vi "Page - Ports.vi"(8 "error in (no error)":errorcluster, 11 "Node Ptr":T3 format="%.0x") -> (0 "error out":errorcluster)   [LabVIEW 2015, in "SLSC-12201 DIO System Explorer.lvlib"]
uses:
  SLSC-12201 DIO System Explorer.lvlib
  <vilib>/NI Veristand/Custom Device API/Custom Device Item Ref.ctl
  <vilib>/Utility/miscctls.llb/LVRowAndColumnTypeDef.ctl
  Direction Control.ctl
  Shared/Constants.vi
  <vilib>/NI Veristand/Custom Device API/Custom Device API.lvlib
  Shared/SLSC-12201 DIO Shared.lvlib
panel:
  in  "Apply":bool
  in  "Port Type":T1 items=["Input", "Output Source", "Output Sink", "Output Push-Pull"]
  out "Cell Position":T2
  in  "Type":u16(ring) items=["Input", "Output Source", "Output Sink", "Output Pull-up"]
  out "Multicolumn Listbox":i32(listbox)=4
  in  "Disable Port":bool
  in  "Enable Port":bool
  in  "SHDocVw.IWebBrowser2":refnum<k7>(container)
  in  "Header":cluster{"Section Name":string}={"Section Name"="Custom Device Item Settings"}
  in  "Description":string
  out "Name":string
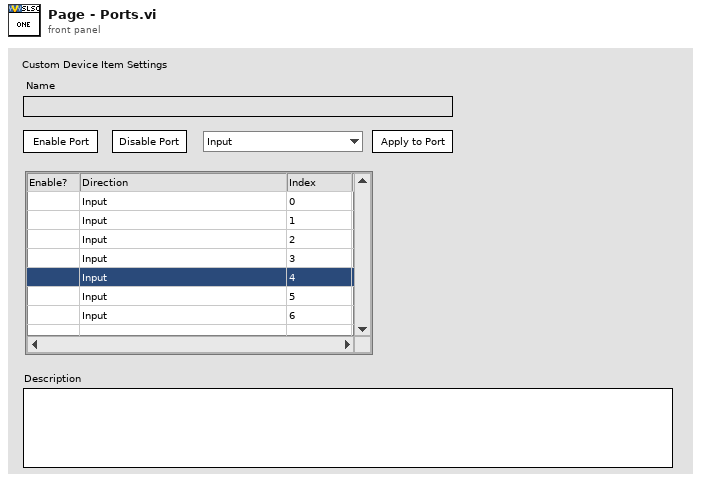
[diagram p1: front panel]
types:
  T1 = typedef "SLSC-12201 DIO System Explorer.lvlib/Direction Control.ctl" = u16
  T2 = typedef "LVRowAndColumnTypeDef.ctl" = cluster{"Row":i32, "Column":i32}
  T3 = typedef "Custom Device API.lvlib/Custom Device Item Ref.ctl" = u64
  T4 = typedef "Custom Device API.lvlib/Custom Device Item Info.ctl" = cluster{"Name":string, "Is Channel":bool, "GUID":string, "Is Waveform":bool}
  T5 = typedef "Custom Device API.lvlib/Custom Device Channel.ctl" = cluster{"Type":T6, "Units":string, "Default Value":dbl, "Faultable":bool, "Scalable":bool}
  T6 = typedef "Custom Device API.lvlib/Custom Device Channel Type.ctl" = enum16{"Input", "Output"}
  T7 = cluster{"Channel Name":string, "SLSC Name":string, "Channel":T5}[]
  T8 = typedef "Custom Device API.lvlib/Custom Device Commands.ctl" = enum16{"Default", "Item renamed", "Shutdown", "Dynamic button pressed"}
  T9 = typedef "LVPoint32TypeDef.ctl" = cluster{"Horizontal":i32, "Vertical":i32}
  T10 = typedef "LVPositionTypeDef.ctl" = cluster{"Left":i32, "Top":i32}
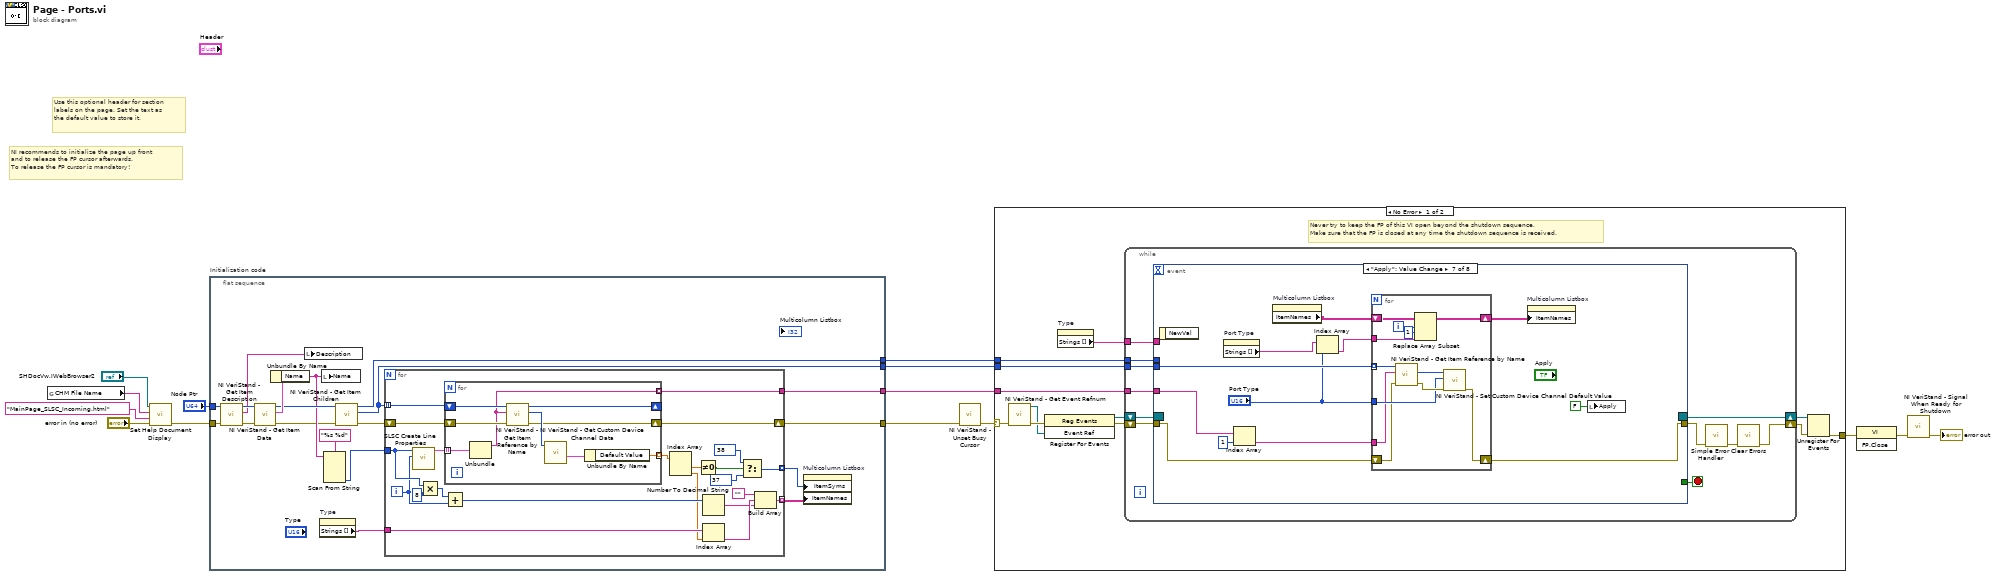
[diagram p0: block diagram]
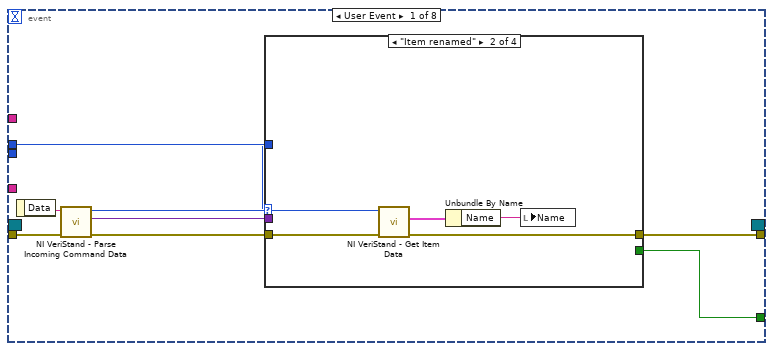
[diagram p2: hidden frame]
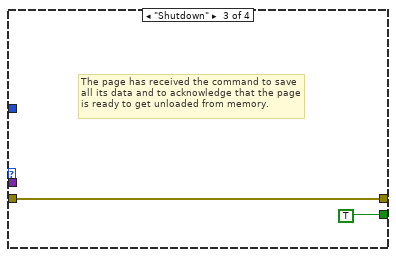
[diagram p4: hidden frame]
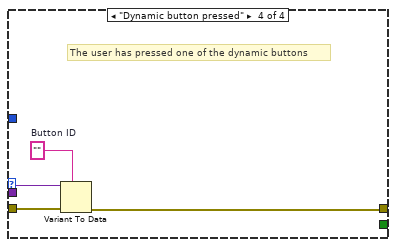
[diagram p5: hidden frame]
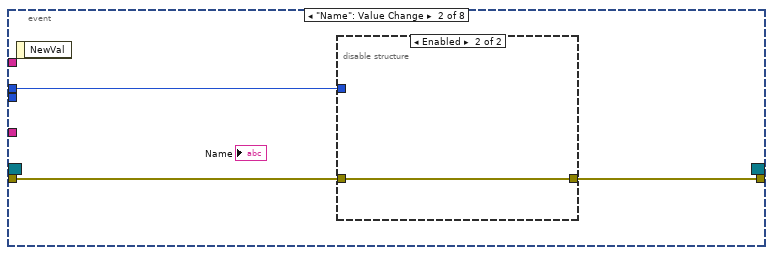
[diagram p6: hidden frame]
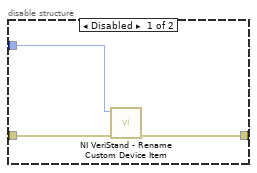
[diagram p7: hidden frame]
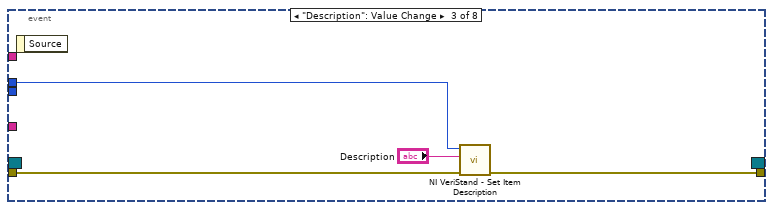
[diagram p8: hidden frame]
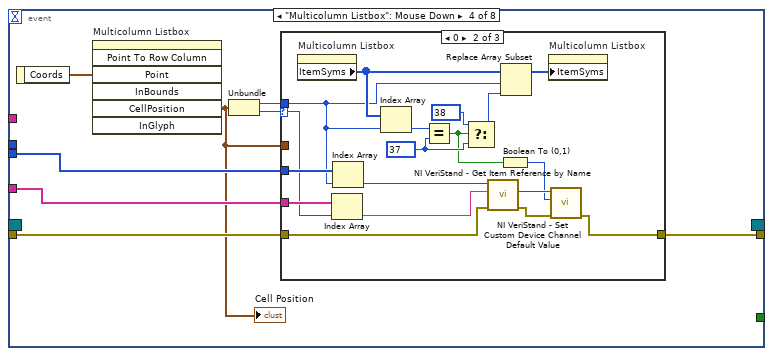
[diagram p9: hidden frame]
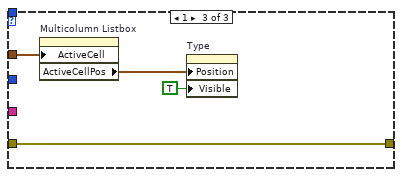
[diagram p11: hidden frame]
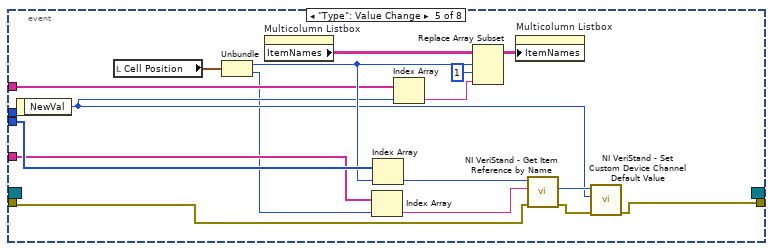
[diagram p12: hidden frame]
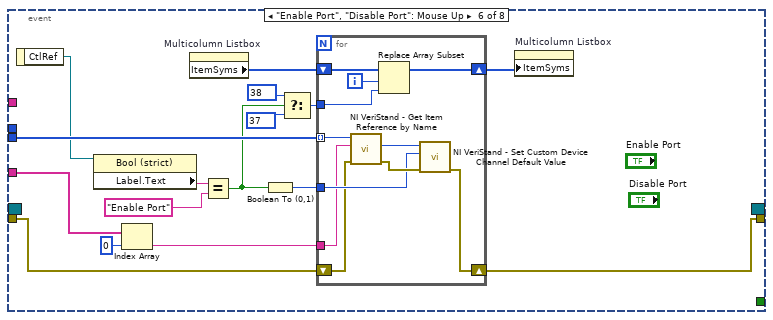
[diagram p13: hidden frame]
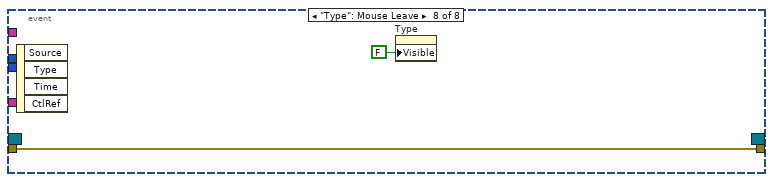
[diagram p14: hidden frame]
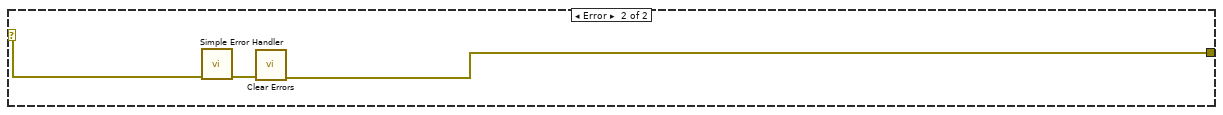
[diagram p15: hidden frame]
diagram:
  # "Use this optional header for section labels on the page. Set the text as the default value to store it."
  # "NI recommends to initialize the page up front\nand to release the FP cursor afterwards.\nTo release the FP cursor is mandatory!"
  n1 = global read "Constants.vi" "CHM File Name"() -> (w3:string)
  n2 = call "Set Help Document Display.vi"("error in (no error)"="error in (no error)", "HTML File"="MainPage_SLSC_Incoming.html", "Main CHM File"=w3, "SHDocVw.IWebBrowser2"="SHDocVw.IWebBrowser2") -> ("error out"=w4:errorcluster)  [unwired: 7 in]
  n3 = flat-sequence "Initialization code" {
    tunnel: w4 -> [w32]
    tunnel: "Node Ptr" -> [w31]
    tunnel: [w27] -> w10
    tunnel: [w25] -> w8
    tunnel: [w21] -> w2
    tunnel: [w20] -> w1
    frame #0 {
      n4 = call <vilib>:"NI VeriStand - Get Item Description.vi"("error in (no error)"=w32, "Item Ref in"=w31) -> ("error out"=w29:errorcluster, "Description"=w30:string, "Item Ref out"=w33:T3)  [unwired: 7 out]
      n5 = call <vilib>:"NI VeriStand - Get Item Data.vi"("error in (no error)"=w29, "Item Ref in"=w33) -> ("error out"=w19:errorcluster, "Item Info"=w28:T4, "Item Ref out"=w26:T3)  [unwired: 7 out]
      n6 = Unbundle By Name(w28) -> ("Name"=w23:string)
      n7 = local write "Description"(w30) -> ()
      n8 = property on="Type" class="Ring (strict)"() -> ("Strings []"=w17:string[])  [unwired: 2 in, 2 out]
      n9 = local write "Name"(w23) -> ()
      n10 = Scan From String(format string="%s %d", input string=w23) -> (output 2=w22:i32)  [unwired: 5 in, 3 out]
      n11 = call <vilib>:"NI VeriStand - Get Item Children.vi"("error in (no error)"=w19, "Item Ref in"=w26) -> ("error out"=w18:errorcluster, "Child Refs"=w21:T3[], "Item Ref out"=w25:T3)  [unwired: 6 in, 1 out]
      n12 = for {
        shift-right: [w54] -> w27
        shift-left: w18 -> [w55]
        tunnel: w21 -> [w51] mode=indexing
        tunnel: w22 -> [w48]
        tunnel: [w49] -> w20
        tunnel: w17 -> [w43]
        tunnel: [w38] -> w16 mode=indexing
        tunnel: [w34] -> w15 mode=indexing
        i -> [w45]
        n13 = call "SLSC Create Line Properties.vi"("Line Number"=w45, "Port Number"=w48) -> ("Outgoing configuration"=w53:T7)  [unwired: 9 in]
        n14 = Multiply(x=w48, y=8) -> (x*y=w46:i32)
        n15 = for {
          shift-right: [w61] -> w54
          shift-left: w55 -> [w62]
          shift-right: [w59] -> _
          shift-left: w51 -> [w60]
          tunnel: w53 -> [w58] mode=indexing
          tunnel: [w57] -> w52 mode=indexing
          tunnel: [w56] -> w49 mode=indexing
          n16 = Unbundle(w58) -> ("Channel Name"=w56:string)  [unwired: 2 out]
          n17 = call <vilib>:"NI VeriStand - Get Item Reference by Name.vi"("error in (no error)"=w62, "Item Name"=w56, "Parent Ref in"=w60) -> ("error out"=w61:errorcluster, "Item Ref"=w64:T3, "Parent Ref out"=w59:T3)  [unwired: 5 in, 1 out]
          n18 = call <vilib>:"NI VeriStand - Get Custom Device Channel Data.vi"("Channel Ref in"=w64) -> ("Channel"=w63:T5)  [unwired: 5 in, 5 out]
          n19 = Unbundle By Name(w63) -> ("Default Value"=w57:dbl)
        }
        n20 = Add(x=w46, y=w45) -> (x+y=w44:i32)
        n21 = Index Array(array=w52) -> (element #1=w50:dbl, element #2=w42:dbl)  [unwired: 2 in]
        n22 = Not Equal To 0?(x=w50) -> (x != 0?=w39:bool)
        n23 = Number To Decimal String(number=w44) -> (decimal integer string=w35:string)  [unwired: 1 in]
        n24 = Index Array(array=w43, index=w42) -> (element=w36:string)
        n25 = Select(t=38, s=w39, f=37) -> (s? t:f=w38:i32)
        n26 = Build Array("", w36, w35) -> (w34:string[])
      }
      n27 = property on="Multicolumn Listbox" class="MCListbox (strict)"("ItemSyms"=w16, "ItemNames"=w15) -> ()  [unwired: 2 in, 2 out]
    }
  }
  n28 = call <vilib>:"NI VeriStand - Unset Busy Cursor.vi"("error in (no error)"=w10) -> ("error out"=w9:errorcluster)  [unwired: 10 out]
  n29 = case shown="No Error" w9 {
    selector: w9 -> [w68 w222]
    tunnel: [w73 w220] -> w14
    tunnel: w8 -> [w69 _]
    tunnel: w2 -> [w67 _]
    tunnel: w1 -> [w66 _]
    frame No Error {
      # "Never try to keep the FP of this VI open beyond the shutdown sequence.\nMake sure that the FP is closed at any time the shutdown sequence is received."
      n30 = call <vilib>:"NI VeriStand - Get Event Refnum.vi"("error in (no error)"=w68) -> ("error out"=w76:errorcluster, "Event Ref"=w72:refnum<user-event>)  [unwired: 9 out]
      n31 = register-events(error in=w76, w72) -> (reference out=w70:refnum<event-registration>, error out=w71:errorcluster)  [unwired: 1 in]
      n32 = property on="Type" class="Ring (strict)"() -> ("Strings []"=w65:string[])  [unwired: 2 in, 2 out]
      n33 = while {
        tunnel: w69 -> [w83]
        shift-right: [w80] -> w74
        shift-left: w71 -> [w86]
        shift-right: [w87] -> w75
        shift-left: w70 -> [w85]
        tunnel: w67 -> [w79]
        tunnel: w66 -> [w78]
        tunnel: w65 -> [w77]
        stop <- w84 stop-if-true
        n34 = event shown="[6] \"Apply\": Value Change" {
          selector: w85 -> [_ _ _ _ _ _ _ _]
          dyn-events: [_ _ _ _ _ _ _ _] -> w87
          timeout: _ -> [_ _ _ _ _ _ _ _]
          tunnel: w86 -> [w95 w110 w117 w121 w153 w172 w201 w219]
          tunnel: [w91 _ _ _ _ _ _ _] -> w84
          tunnel: [w90 w109 w116 w120 w151 w171 w200 w219] -> w82
          tunnel: w83 -> [w89 w108 w118 _ _ _ _ _]
          tunnel: w79 -> [_ _ _ w123 w157 w182 w205 _]
          tunnel: w78 -> [_ _ _ w122 w156 w175 w204 _]
          tunnel: w77 -> [_ _ _ _ w152 _ _ _]
          event User Event {
            n35 = event-data() -> ("Data"=w94:string)  [unwired: 1 out]
            n36 = call <vilib>:"NI VeriStand - Parse Incoming Command Data.vi"("error in (no error)"=w95, "Incoming data"=w94) -> ("error out"=w93:errorcluster, "Outgoing data"=w88:variant, "Action"=w92:T8)  [unwired: 7 out]
            n37 = case shown="\"Item renamed\"" w92 {
              tunnel: w93 -> [w96 w101 w102 w107]
              tunnel: [_ _ TRUE _] -> w91
              tunnel: [w96 w98 w102 w104] -> w90
              tunnel: w89 -> [_ w100 _ _]
              tunnel: w88 -> [_ _ _ w106]
              frame "Default", Default {
              }
              frame "Item renamed" {
                n38 = call <vilib>:"NI VeriStand - Get Item Data.vi"("error in (no error)"=w101, "Item Ref in"=w100) -> ("error out"=w98:errorcluster, "Item Info"=w99:T4)  [unwired: 8 out]
                n39 = Unbundle By Name(w99) -> ("Name"=w97:string)
                n40 = local write "Name"(w97) -> ()
              }
              frame "Shutdown" {
                # "The page has received the command to save all its data and to acknowledge that the page is ready to get unloaded from memory."
              }
              frame "Dynamic button pressed" {
                w105 = ""  # Button ID
                # "The user has pressed one of the dynamic buttons"
                n41 = Variant To Data(error in=w107, type=w105, Variant=w106) -> (error out=w104:errorcluster)  [unwired: 1 out]
              }
            }
          }
          event "Name": Value Change {
            n42 = event-data() -> ()  [unwired: 2 out]
            n43 = disable-structure shown="Enabled" {
              disable-tunnel: w110 -> [w113 w114]
              disable-tunnel: [w112 w114] -> w109
              disable-tunnel: w108 -> [w111 _]
              frame Disabled {
                n44 = call <vilib>:"NI VeriStand - Rename Custom Device Item.vi"("error in (no error)"=w113, "Item Ref in"=w111) -> ("error out"=w112:errorcluster)  [unwired: 2 in, 7 out]
              }
              frame Enabled {
              }
            }
          }
          event "Description": Value Change {
            n45 = event-data() -> ()  [unwired: 2 out]
            n46 = call <vilib>:"NI VeriStand - Set Item Description.vi"("error in (no error)"=w117, "Description"="Description", "Item Ref in"=w118) -> ("error out"=w116:errorcluster)  [unwired: 8 out]
          }
          event "Multicolumn Listbox": Mouse Down {
            n47 = event-data() -> ("Coords"=w126:T9)  [unwired: 1 out]
            n48 = invoke on="Multicolumn Listbox" class="MCListbox (strict)" method="Point To Row Column"("Point"=w126) -> ("CellPosition"=w119:T2)  [unwired: 6 in, 6 out]
            "Cell Position" <- w119
            n49 = Unbundle(w119) -> ("Row"=w124:i32, "Column"=w125:i32)
            n50 = case shown="0" w125 {
              selector: w125 -> [_ w128 _]
              tunnel: w124 -> [_ w134 _]
              tunnel: w123 -> [_ w139 _]
              tunnel: w122 -> [_ w135 _]
              tunnel: w121 -> [w127 w130 w146]
              tunnel: [w127 w129 w146] -> w120
              tunnel: w119 -> [_ _ w149]
              frame 2, Default {
              }
              frame 0 {
                w144 = 37
                n51 = property on="Multicolumn Listbox" class="MCListbox (strict)"() -> ("ItemSyms"=w141:i32[])  [unwired: 2 in, 2 out]
                n52 = Index Array(array=w135, index=w128) -> (element=w133:string)
                n53 = Index Array(array=w139, index=w134) -> (element=w136:T3)
                n54 = Index Array(array=w141, index=w134) -> (element=w143:i32)
                n55 = Equal?(x=w143, y=w144) -> (x = y?=w132:bool)
                n56 = Select(t=38, s=w132, f=w144) -> (s? t:f=w142:i32)
                n57 = call <vilib>:"NI VeriStand - Get Item Reference by Name.vi"("error in (no error)"=w130, "Item Name"=w133, "Parent Ref in"=w136) -> ("error out"=w138:errorcluster, "Item Ref"=w137:T3)  [unwired: 5 in, 2 out]
                n58 = Boolean To (0,1)(Boolean=w132) -> (0, 1=w131:i16)
                n59 = Replace Array Subset(array=w141, new element=w142, index=w134) -> (w140:i32[])
                n60 = property on="Multicolumn Listbox" class="MCListbox (strict)"("ItemSyms"=w140) -> ()  [unwired: 2 in, 2 out]
                n61 = call <vilib>:"NI VeriStand - Set Custom Device Channel Default Value.vi"("error in (no error)"=w138, "Default Value"=w131, "Channel Ref in"=w137) -> ("error out"=w129:errorcluster)  [unwired: 7 in, 1 out]
              }
              frame 1 {
                n62 = property on="Multicolumn Listbox" class="MCListbox (strict)"("ActiveCell"=w149) -> ("ActiveCellPos"=w148:T10)  [unwired: 2 in, 2 out]
                n63 = property on="Type" class="Ring (strict)"("Position"=w148, "Visible"=TRUE) -> ()  [unwired: 2 in, 2 out]
              }
            }
          }
          event "Type": Value Change {
            n64 = event-data() -> ("NewVal"=w154:u16)  [unwired: 1 out]
            n65 = local read "Cell Position"() -> (w163:T2)
            n66 = Unbundle(w163) -> ("Row"=w155:i32, "Column"=w150:i32)
            n67 = property on="Multicolumn Listbox" class="MCListbox (strict)"() -> ("ItemNames"=w166:string[][])  [unwired: 2 in, 2 out]
            n68 = Index Array(array=w156, index=w150) -> (element=w158:string)
            n69 = Index Array(array=w157, index=w155) -> (element=w159:T3)
            n70 = Index Array(array=w152, index=w154) -> (element=w162:string)
            n71 = Replace Array Subset(array=w166, new element=w162, index (row)=w155, index (col)=1 ("disabled index (col)")) -> (w165:string[][])
            n72 = property on="Multicolumn Listbox" class="MCListbox (strict)"("ItemNames"=w165) -> ()  [unwired: 2 in, 2 out]
            n73 = call <vilib>:"NI VeriStand - Get Item Reference by Name.vi"("error in (no error)"=w153, "Item Name"=w158, "Parent Ref in"=w159) -> ("error out"=w161:errorcluster, "Item Ref"=w160:T3)  [unwired: 5 in, 2 out]
            n74 = call <vilib>:"NI VeriStand - Set Custom Device Channel Default Value.vi"("error in (no error)"=w161, "Default Value"=w154, "Channel Ref in"=w160) -> ("error out"=w151:errorcluster)  [unwired: 7 in, 1 out]
          }
          event "Enable Port", "Disable Port": Mouse Up {
            n75 = event-data() -> ("CtlRef"=w179:refnum<vi>)  [unwired: 1 out]
            n76 = property class="Bool (strict)"(reference=w179) -> ("Label.Text"=w178:string)  [unwired: 1 in, 2 out]
            n77 = Index Array(array=w175, index=0) -> (element=w173:string)
            n78 = property on="Multicolumn Listbox" class="MCListbox (strict)"() -> ("ItemSyms"=w181:i32[])  [unwired: 2 in, 2 out]
            n79 = Equal?(x=w178, y="Enable Port") -> (x = y?=w170:bool)
            n80 = Boolean To (0,1)(Boolean=w170) -> (0, 1=w176:i16)
            n81 = Select(t=38, s=w170, f=37) -> (s? t:f=w167:i32)
            n82 = for {
              tunnel: w182 -> [w191] mode=indexing
              shift-right: [w188] -> w180
              shift-left: w181 -> [w189]
              tunnel: w176 -> [w187]
              tunnel: w173 -> [w186]
              shift-right: [w184] -> w171
              shift-left: w172 -> [w185]
              tunnel: w167 -> [w183]
              i -> [w190]
              n83 = call <vilib>:"NI VeriStand - Get Item Reference by Name.vi"("error in (no error)"=w185, "Item Name"=w186, "Parent Ref in"=w191) -> ("error out"=w193:errorcluster, "Item Ref"=w192:T3)  [unwired: 5 in, 2 out]
              n84 = Replace Array Subset(array=w189, new element=w183, index=w190) -> (w188:i32[])
              n85 = call <vilib>:"NI VeriStand - Set Custom Device Channel Default Value.vi"("error in (no error)"=w193, "Default Value"=w187, "Channel Ref in"=w192) -> ("error out"=w184:errorcluster)  [unwired: 7 in, 1 out]
            }
            n86 = property on="Multicolumn Listbox" class="MCListbox (strict)"("ItemSyms"=w180) -> ()  [unwired: 2 in, 2 out]
          }
          event "Apply": Value Change {
            n87 = event-data() -> ()  [unwired: 2 out]
            n88 = property on="Port Type" class="Ring (strict)"() -> ("Strings []"=w197:string[])  [unwired: 2 in, 2 out]
            n89 = Index Array(array=w204, index=1) -> (element=w202:string)
            n90 = property on="Multicolumn Listbox" class="MCListbox (strict)"() -> ("ItemNames"=w199:string[][])  [unwired: 2 in, 2 out]
            n91 = Index Array(array=w197, index="Port Type") -> (element=w195:string)
            n92 = for {
              tunnel: w205 -> [w215] mode=indexing
              shift-right: [w212] -> w198
              shift-left: w199 -> [w213]
              tunnel: "Port Type" -> [w211]
              tunnel: w202 -> [w210]
              shift-right: [w208] -> w200
              shift-left: w201 -> [w209]
              tunnel: w195 -> [w206]
              i -> [w214]
              n93 = call <vilib>:"NI VeriStand - Get Item Reference by Name.vi"("error in (no error)"=w209, "Item Name"=w210, "Parent Ref in"=w215) -> ("error out"=w217:errorcluster, "Item Ref"=w216:T3)  [unwired: 5 in, 2 out]
              n94 = Replace Array Subset(array=w213, new element=w206, index (row)=w214, index (col)=1 ("disabled index (col)")) -> (w212:string[][])
              n95 = call <vilib>:"NI VeriStand - Set Custom Device Channel Default Value.vi"("error in (no error)"=w217, "Default Value"=w211, "Channel Ref in"=w216) -> ("error out"=w208:errorcluster)  [unwired: 7 in, 1 out]
            }
            n96 = property on="Multicolumn Listbox" class="MCListbox (strict)"("ItemNames"=w198) -> ()  [unwired: 2 in, 2 out]
            n97 = local write "Apply"(FALSE ("Apply")) -> ()
          }
          event "Type": Mouse Leave {
            n98 = event-data() -> ()  [unwired: 5 out]
            n99 = property on="Type" class="Ring (strict)"("Visible"=FALSE) -> ()  [unwired: 2 in, 2 out]
          }
        }
        n100 = call <vilib>:"Simple Error Handler.vi"("error in (no error)"=w82) -> ("error out"=w81:errorcluster)  [unwired: 1 in, 7 out]
        n101 = call <vilib>:"Clear Errors.vi"("error in (no error)"=w81) -> ("error out"=w80:errorcluster)  [unwired: 1 in, 5 out]
      }
      n102 = Unregister For Events(event registration refnum=w75, error in=w74) -> (error out=w73:errorcluster)
    }
    frame Error {
      n103 = call <vilib>:"Simple Error Handler.vi"("error in (no error)"=w222) -> ("error out"=w221:errorcluster)  [unwired: 1 in, 7 out]
      n104 = call <vilib>:"Clear Errors.vi"("error in (no error)"=w221) -> ("error out"=w220:errorcluster)  [unwired: 1 in, 5 out]
    }
  }
  n105 = invoke class="VI" method="FP.Close"(error in=w14) -> (error out=w13:errorcluster)  [unwired: 2 in, 2 out]
  n106 = call <vilib>:"NI VeriStand - Signal When Ready for Shutdown.vi"("error in (no error)"=w13) -> ("error out"=→"error out":errorcluster)  [unwired: 10 out]
